vi "Read CAN FIFO.vi"(8 "error in (no error)":errorcluster, 9 "Timeout (ms)":i32, 11 "CIFTag in":refnum<class "CIFFifoCAN.lvclass">) -> (0 "error out":errorcluster, 1 "timed out?":bool, 2 "Data":T2 {"payload" format="%x"; "identifier" format="%x"}, 3 "CIFTag out":refnum<class "CIFFifoCAN.lvclass">, 4 "Header":T1)   [LabVIEW 2021, in "CIFFifoCAN.lvclass"]
uses:
  CIFFifoCAN.lvclass
  D:/dev/CIF-LVCore/src/Channels/CIFChannels/CIFChannels.lvclass
  D:/dev/CIF-LVCore/src/Channels/CIFTag/CIFTag/CIFTag.lvclass
  ChannelRegistrar/typedef/Datatype CAN.ctl
  ChannelCommon/typedef/FIFO Header.ctl
  CIFChannels/CIFChannels.lvclass/CIFChannels.ctl
  CIFChannels/Typedef/Channel State.ctl
  CIFChannels/Typedef/Direction.ctl
  CIFTag/CIFTag.lvclass/CIFTag.ctl
  CIFFifoCAN.lvclass/CIFFifoCAN.ctl
  CIFFIFO/CIFfifo.lvclass/CIFfifo.ctl
  CIFChannels/Accessors/Read Channel State.vi
  CIFChannels/Accessors/Read Direction.vi
  CIFChannels/Accessors/Write Channel State.vi
  CIFChannels/Accessors/Read Disconnect Behavior.vi
  <vilib>/CIFChannels/Top Level/Read Variable Length U8 Array.vi/81056090-23cf-424a-a716-29db01c8ef1b.vi
  <vilib>/CIFChannels/Top Level/Read Variable Length U8 Array.vi/6610cd62-0a6d-4591-8fd4-6453482a4bc1.vi
  <vilib>/CIFChannels/Top Level/Read Variable Length U8 Array.vi/93d598b0-524b-4f76-9570-a74a86ef2c6f.vi
  CIFFIFO/Accessors/Write Timeout.vi
  ChannelCommon/Utilities/Unflatten Header.vi
  CIFFIFO/Accessors/Read Header.vi
  CIFFIFO/Accessors/Write Header.vi
  <vilib>/CIFChannels/Top Level/Read Variable Length U8 Array.vi/81056090-23cf-424a-a716-29db01c8ef1b.vi/4bc1c15b-36ab-481f-b8dd-c64075ce723a.vi
  <vilib>/CIFChannels/Top Level/Read Variable Length U8 Array.vi/81056090-23cf-424a-a716-29db01c8ef1b.vi/d83cb72b-7713-41fc-a3d1-682de79cf574.vi
  <vilib>/CIFChannels/SubVIs/Get dll Path.vi
  <vilib>/CIFChannels/Top Level/Read Variable Length U8 Array.vi/6610cd62-0a6d-4591-8fd4-6453482a4bc1.vi/c28b0ead-42ad-4072-80a2-aca7f2bd7ce3.vi
  <vilib>/CIFChannels/Top Level/Read Variable Length U8 Array.vi/93d598b0-524b-4f76-9570-a74a86ef2c6f.vi/4bc1c15b-36ab-481f-b8dd-c64075ce723a.vi
  <vilib>/CIFChannels/Top Level/Read Variable Length U8 Array.vi/93d598b0-524b-4f76-9570-a74a86ef2c6f.vi/d83cb72b-7713-41fc-a3d1-682de79cf574.vi
  CIFTag/CIFTag.lvclass
  CIFChannels/CIFChannels.lvclass
  <vilib>/CIFChannels/CIFChannelCore.lvlib
  ChannelRegistrar/ChannelRegistrar.lvlib
  ChannelCommon/ChannelCommon.lvlib
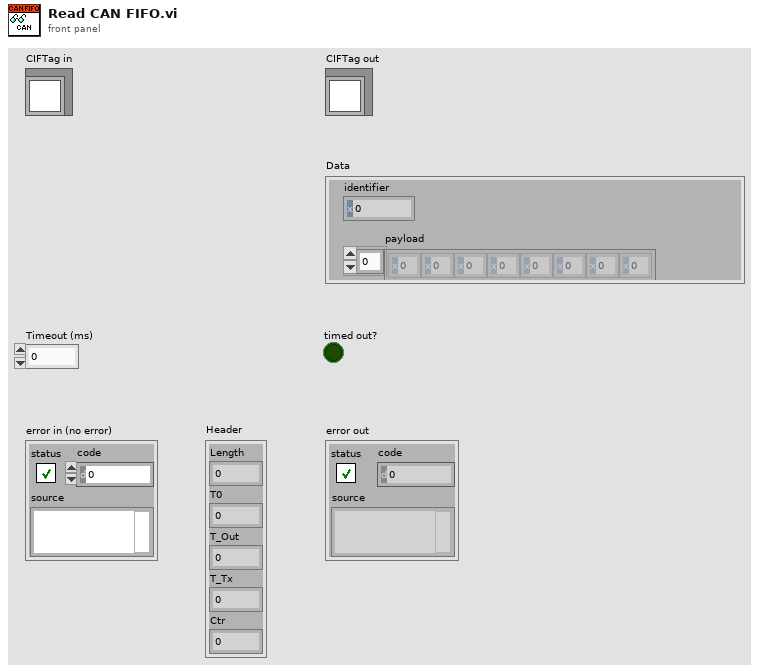
[diagram p1: front panel]
types:
  T1 = typedef "ChannelCommon.lvlib/FIFO Header.ctl" = cluster{"Length":u64, "T0":u64, "T_Out":u64, "T_Tx":u64, "Ctr":u64}
  T2 = typedef "ChannelRegistrar.lvlib/Datatype CAN.ctl" = cluster{"payload":u8[], "identifier":u32}
  T3 = typedef "CIFChannels.lvclass/Channel State.ctl" = enum16{"Creating", "Disconnected", "Connecting", "Connected", "Destroyed"}
  T4 = typedef "CIFChannels.lvclass/Direction.ctl" = enum16{"Publisher", "Subscriber"}
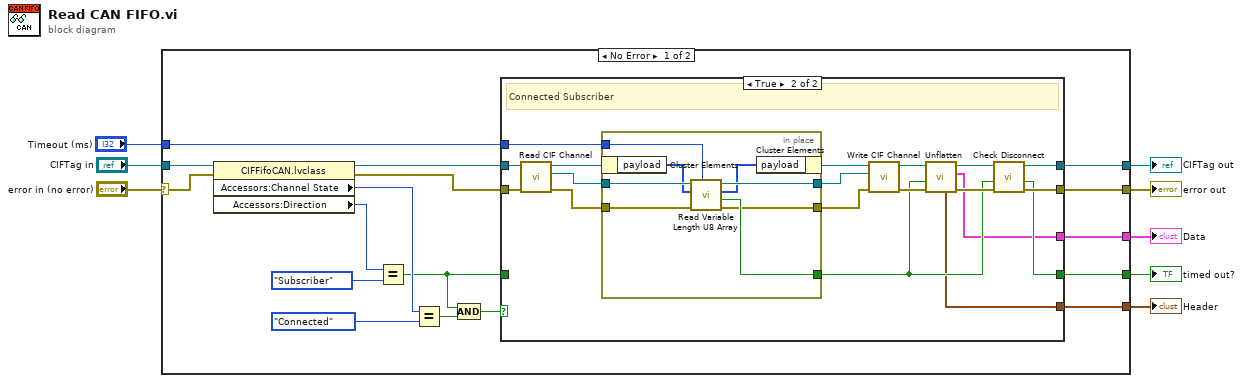
[diagram p0: block diagram]
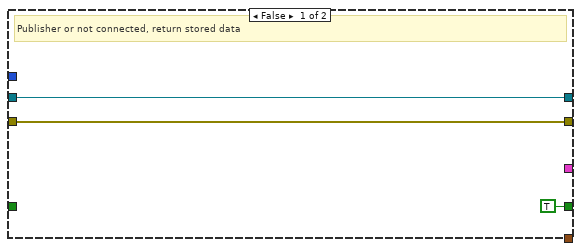
[diagram p2: hidden frame]
diagram:
  n1 = case shown="No Error" "error in (no error)" {
    selector: "error in (no error)" -> [w22 w57]
    tunnel: [w11 w57] -> w7
    tunnel: [w12 w56] -> w5
    tunnel: "CIFTag in" -> [w23 w56]
    tunnel: [w25 _] -> w4
    tunnel: [w24 _] -> w2
    tunnel: "Timeout (ms)" -> [w10 _]
    tunnel: [w9 _] -> w1
    frame No Error {
      n2 = property class="CIFFifoCAN.lvclass"(reference=w23, error in=w22) -> (reference out=w21:refnum<class "CIFFifoCAN.lvclass">, error out=w20:errorcluster, "Accessors:Channel State"=w17:T3, "Accessors:Direction"=w19:T4)
      n3 = Equal?(x=w19, y=Direction."Subscriber") -> (x = y?=w13:bool)
      n4 = Equal?(x=w17, y=Channel_State."Connected") -> (x = y?=w15:bool)
      n5 = Compound Arithmetic op=AND(w13, w15) -> (w14:bool)
      n6 = case shown="True" w14 {
        tunnel: [TRUE ("timeout out") w37] -> w25
        tunnel: [_ w30] -> w24
        tunnel: w20 -> [w27 w46]
        tunnel: w21 -> [w28 w47]
        tunnel: w13 -> [_ _]
        tunnel: [w28 w45] -> w12
        tunnel: [w27 w44] -> w11
        tunnel: w10 -> [_ w36]
        tunnel: [_ w29] -> w9
        frame False {
          # "Publisher or not connected, return stored data"
        }
        frame True {
          # "Connected Subscriber"
          n7 = call "Read CIF Channel.vi"("error in (no error)"=w46, "CIFTag in"=w47) -> ("error out"=w41:errorcluster, "CIF Channel"=w42:refnum<k21>, "CIFTag out"=w43:refnum<class "CIFFifoCAN.lvclass">)  [unwired: 7 in]
          n8 = in-place {
            in-place-border: [w53] -> w31
            in-place-border: w42 -> [w55]
            in-place-border: w41 -> [w54]
            in-place-border: [w52] -> w38
            in-place-border: [w51] -> w39
            in-place-border: w36 -> [w50]
            n9 = in-place-cluster #1(w43) -> ("payload"=w49:u8[])
            n10 = call <vilib>:"Read Variable Length U8 Array.vi"("Timeout (ms)"=w50, "error in"=w54, "Payload in"=w49, "CIF Channel in"=w55) -> ("error out"=w51:errorcluster, "Timed out?"=w53:bool, "Payload out"=w48:u8[], "CIF Channel out"=w52:refnum<k21>)  [unwired: 4 in]
            n11 = in-place-cluster #1("payload"=w48) -> (w40:refnum<class "CIFFifoCAN.lvclass">)
          }
          n12 = call "Write CIF Channel.vi"("error in (no error)"=w39, "CIF Channel"=w38, "CIFTag in"=w40) -> ("error out"=w34:errorcluster, "CIFTag out"=w35:refnum<class "CIFFifoCAN.lvclass">)  [unwired: 7 in]
          n13 = call "Unflatten.vi"("error in (no error)"=w34, "timeout in"=w31, "CIFFifoCAN in"=w35) -> ("error out"=w32:errorcluster, "Data"=w30:T2, "CIFFifoCAN out"=w33:refnum<class "CIFFifoCAN.lvclass">, "Header"=w29:T1)  [unwired: 5 in]
          n14 = call "Check Disconnect.vi"("error in (no error)"=w32, "timeout in"=w31, "CIFTag in"=w33) -> ("error out"=w44:errorcluster, "timeout out"=w37:bool, "CIFTag out"=w45:refnum<class "CIFFifoCAN.lvclass">)  [unwired: 5 in, 1 out]
        }
      }
    }
    frame Error {
    }
  }
  "error out" <- w7
  "CIFTag out" <- w5
  "timed out?" <- w4
  "Data" <- w2
  "Header" <- w1
